vi "Operaciones Numericas.vi"() -> ()   [LabVIEW 2020]
panel:
  out "Resultado Divicion":dbl
  out "Resultado Multiplicacion":dbl
  out "Resultado Resta":dbl
  in  "Dato 5":dbl(slide) scale=0.0..10.0
  out "Resultado Suma":dbl
  in  "Dato 4":dbl(slide) scale=0.0..10.0
  in  "Dato 3":dbl(slide) scale=0.0..10.0
  in  "Dato 2":dbl(slide) scale=0.0..10.0
  in  "Dato 1":dbl(slide) scale=0.0..10.0
  # "Operaciones Numericas"
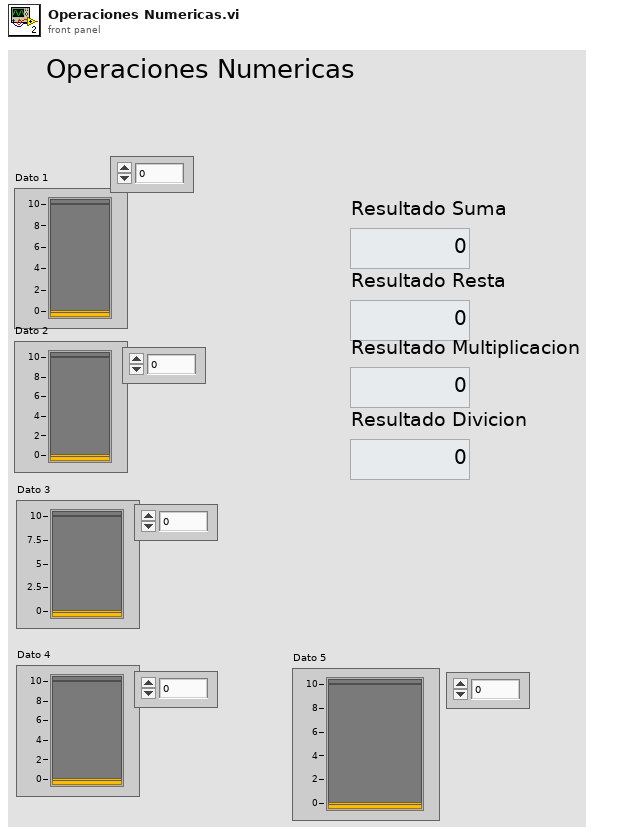
[diagram p1: front panel]
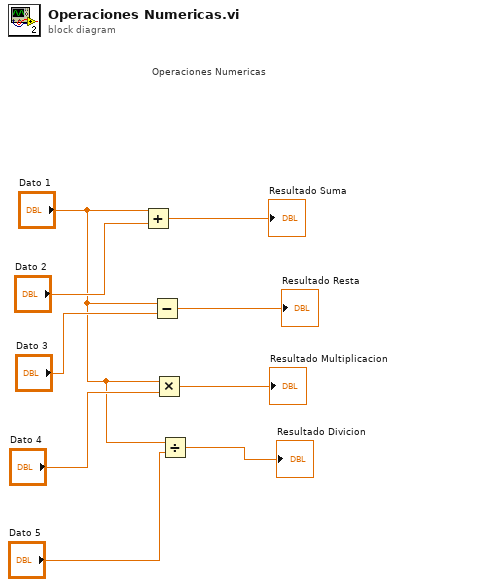
[diagram p0: block diagram]
diagram:
  # "Operaciones Numericas"
  n1 = Add(x="Dato 1", y="Dato 2") -> (x+y=→"Resultado Suma":dbl)
  n2 = Subtract(x="Dato 1", y="Dato 3") -> (x-y=→"Resultado Resta":dbl)
  n3 = Multiply(x="Dato 1", y="Dato 4") -> (x*y=→"Resultado Multiplicacion":dbl)
  n4 = Divide(x="Dato 1", y="Dato 5") -> (x/y=→"Resultado Divicion":dbl)
